vi "CanChannelRead.vi"() -> ()   [LabVIEW 2012]
panel:
  out "error out":errorcluster {"code" format="%.0x"}
  out "Update":u32 format="%010.0f"
  in  "TX Threshold":u16=1
  in  "RX Threshold":u16=1
  out "Channel Status":T1 {"TX Load (%)" max=100 scale=0.0..100.0; "RX Load (%)" max=100 scale=0.0..100.0; "Line Status"."BUS Timing"."BTR1" format="%02x"; "Line Status"."BUS Timing"."BTR0" format="%02x"; "Line Status"."BUS Load (%)" max=100 step=1 scale=0.0..100.0}
  in  "Stop":bool
  in  "Activate":bool
  in  "TX FIFO Size":u16=16
  in  "RX FIFO Size":u16=128
  in  "Exclusive":bool
  out "Message Count":u32
  out "CAN message":T2 {"Data"."[4]" format="%02x"; "Data"."[7]" format="%02x"; "Data"."[6]" format="%02x"; "Data"."[5]" format="%02x"; "Data"."[3]" format="%02x"; "Data"."[2]" format="%02x"; "Data"."[1]" format="%02x"; "Data"."[0]" format="%02x"; "Timestamp" format="%08x"; "Arbitration ID" format="%08x"}
  out "IsRunning":bool
  # "Channel Configuration"
  # "Channel Status"
  # "CAN message"
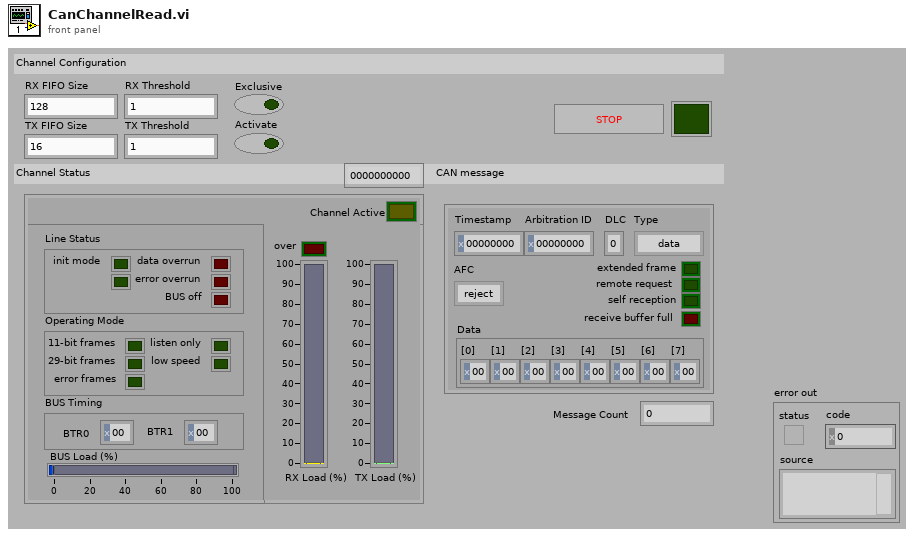
[diagram p1: front panel]
types:
  T1 = cluster{"Line Status":cluster{"Line Status":cluster{"init mode":bool, "TX pending":bool, "data overrun":bool, "error overrun":bool, "BUS off":bool}, "Operating Mode":cluster{"11-bit frames":bool, "29-bit frames":bool, "error frames":bool, "listen only":bool, "low speed":bool}, "BUS Timing":cluster{"BTR0":u8, "BTR1":u8}, "BUS Load (%)":u8}, "Channel Active":bool, "over":bool, "RX Load (%)":u8, "TX Load (%)":u8}
  T2 = cluster{"Timestamp":u32, "Arbitration ID":u32, "DLC":u8, "Type":enum8{"data", "info", "error", "status", "wakeup", "timer ovr", "timer reset"}, "AFC":enum8{"reject", "always", "filter 1", "filter 2"}, "extended frame":bool, "remote request":bool, "self reception":bool, "receive buffer full":bool, "Data":cluster{"[0]":u8, "[1]":u8, "[2]":u8, "[3]":u8, "[4]":u8, "[5]":u8, "[6]":u8, "[7]":u8}}
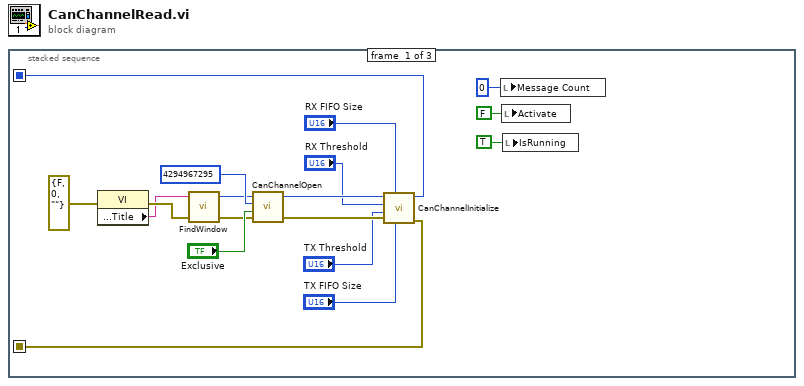
[diagram p0: block diagram]
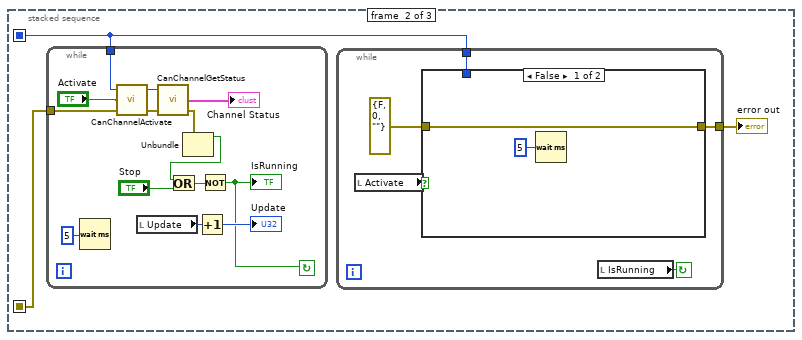
[diagram p2: hidden frame]
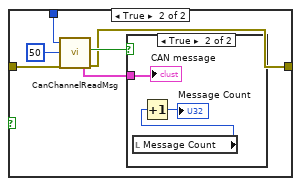
[diagram p3: hidden frame]
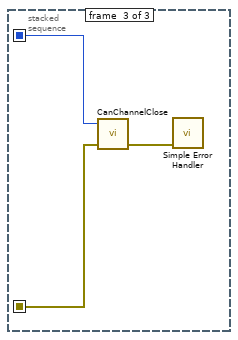
[diagram p5: hidden frame]
diagram:
  n1 = stacked-sequence {
    seq-local: [w14 _ _] -> [_ w20 w54]
    seq-local: [w7 _ _] -> [_ w21 w52]
    frame #0 {
      n2 = property class="VI"(error in=errorcluster {"status"=FALSE, "code"=0, "source"=""}) -> (error out=w3:errorcluster, "Front Panel Window:Title"=w2:string)  [unwired: 1 in, 1 out]
      n3 = call "FindWindow.vi"("error in"=w3, "Window Title"=w2) -> ("error out"=w4:errorcluster, "HWND"=w5:u32)  [unwired: 2 in]
      n4 = call "CanChannelOpen.vi"("error in"=w4, "Exclusive"="Exclusive", "CAN Number"=u32 4294967295, "Device Handle"=w5) -> ("error out"=w16:errorcluster, "CAN Channel Handle"=w15:u32)  [unwired: 1 in]
      n5 = call "CanChannelInitialize.vi"("TX Fifo Size"="TX FIFO Size", "RX Fifo Size"="RX FIFO Size", "error in"=w16, "TX Threshold"="TX Threshold", "RX Threshold"="RX Threshold", "CAN Channel Handle in"=w15) -> ("error out"=w7:errorcluster, "CAN Channel Handle out"=w14:u32)  [unwired: 1 in, 1 out]
      n6 = local write "Message Count"(u32 0 ("Message Count")) -> ()
      n7 = local write "Activate"(FALSE ("Activate")) -> ()
      n8 = local write "IsRunning"(TRUE ("IsRunning")) -> ()
    }
    frame #1 {
      n9 = while {
        tunnel: w20 -> [w48]
        tunnel: w21 -> [w47]
        stop <- w38 continue-if-true
        n10 = Wait (ms)(milliseconds to wait=u32 5) -> ()  [unwired: 1 out]
        n11 = call "CanChannelActivate.vi"("error in"=w47, "activate"="Activate", "CAN Channel Handle in"=w48) -> ("error out"=w50:errorcluster, "CAN Channel Handle out"=w49:u32)  [unwired: 1 out]
        n12 = local read "Update"() -> (w40:u32)
        n13 = call "CanChannelGetStatus.vi"("error in"=w50, "CAN Channel Handle in"=w49) -> ("error out"=w46:errorcluster, "Channel Status"=→"Channel Status":T1)  [unwired: 1 in, 1 out]
        n14 = Unbundle(w46) -> ("status"=w45:bool)  [unwired: 2 out]
        n15 = Or(x=w45, y="Stop") -> (x .or. y?=w44:bool)
        n16 = Increment(x=w40) -> (x+1=→"Update":u32)
        n17 = Not(x=w44) -> (.not. x?=w38:bool)
        "IsRunning" <- w38
      }
      n18 = while {
        tunnel: w20 -> [w25]
        tunnel: [w23] -> w19
        stop <- w26 continue-if-true
        n19 = local read "Activate"() -> (w24:bool)
        n20 = case shown="False" w24 {
          tunnel: w25 -> [_ w33]
          tunnel: [w27 w30] -> w23
          tunnel: errorcluster {"status"=FALSE, "code"=0, "source"=""} ("error in") -> [w27 w29]
          frame False {
            n21 = Wait (ms)(milliseconds to wait=u32 5) -> ()  [unwired: 1 out]
          }
          frame True {
            n22 = call "CanChannelReadMsg.vi"("CAN Channel Handle in"=w33, "Milliseconds"=u32 50, "error in"=w29) -> ("Is Valid Message"=w32:bool, "CAN message"=w31:T2, "error out"=w30:errorcluster)  [unwired: 1 out]
            n23 = case shown="True" w32 {
              tunnel: w31 -> [_ w35]
              frame False {
              }
              frame True {
                n24 = local read "Message Count"() -> (w37:u32)
                n25 = Increment(x=w37) -> (x+1=→"Message Count":u32)
                "CAN message" <- w35
              }
            }
          }
        }
        n26 = local read "IsRunning"() -> (w26:bool)
      }
      "error out" <- w19
    }
    frame #2 {
      n27 = call "CanChannelClose.vi"("error in"=w52, "CAN Channel Handle"=w54) -> ("error out"=w53:errorcluster)  [unwired: 3 in]
      n28 = call <vilib>:"Simple Error Handler.vi"("error in (no error)"=w53) -> ()  [unwired: 4 in, 5 out]
    }
  }
